vi "Close RxTx.vi"(8 "error in (no error)":errorcluster, 11 "Filter_Wheel in":refnum<class "Filter_Wheel.lvclass">) -> (0 "error out":errorcluster, 3 "Filter_Wheel out":refnum<class "Filter_Wheel.lvclass">)   [LabVIEW 2018, in "Filter_Wheel.lvclass"]
uses:
  Filter_Wheel.lvclass
  Filter_Wheel.lvclass/Filter_Wheel.ctl
  RxTx/RxTx.lvclass
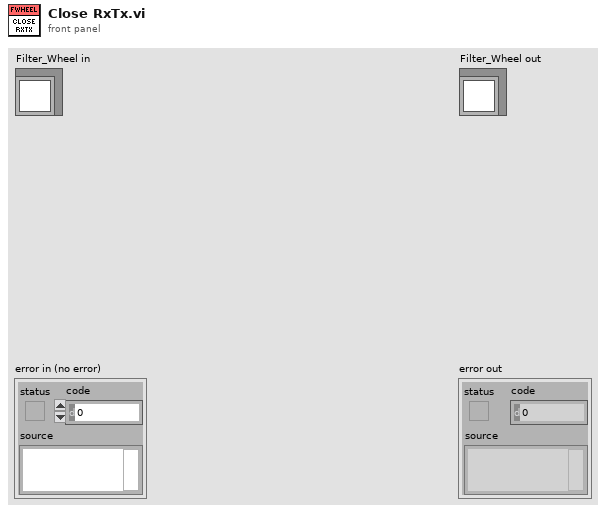
[diagram p1: front panel]
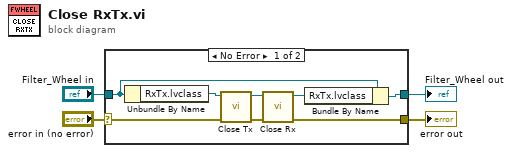
[diagram p0: block diagram]
diagram:
  n1 = case shown="No Error" "error in (no error)" {
    selector: "error in (no error)" -> [w12 w14]
    tunnel: [w10 w14] -> w3
    tunnel: [w8 w13] -> w1
    tunnel: "Filter_Wheel in" -> [w9 w13]
    frame No Error {
      n2 = Unbundle By Name(w9) -> ("RxTx.lvclass"=w5:refnum<class "RxTx.lvclass">)
      n3 = call "Close Tx.vi"("error in (no error)"=w12, "RxTx in"=w5) -> ("error out"=w11:errorcluster, "RxTx out"=w6:refnum<class "RxTx.lvclass">)  [unwired: 8 in]
      n4 = call "Close Rx.vi"("error in (no error)"=w11, "RxTx in"=w6) -> ("error out"=w10:errorcluster, "RxTx out"=w7:refnum<class "RxTx.lvclass">)  [unwired: 8 in]
      n5 = Bundle By Name(cluster=w9, "RxTx.lvclass"=w7) -> (w8:refnum<class "Filter_Wheel.lvclass">)
    }
    frame Error {
    }
  }
  "error out" <- w3
  "Filter_Wheel out" <- w1
